vi "Utils - Convert1DImageToLVImage.vi"(6 "picture":picture, 8 "error in (no error)":errorcluster, 9 "1DImageData In":u8[](array[numeric]), 11 "Image Properties In":T1) -> (0 "error out":errorcluster, 1 "1DImageData Out":u8[](array[numeric]), 4 "new picture":picture)   [LabVIEW 2015]
doc: "Convert 1d U8 Image array to LabVIEW image. This VI supports only Mono8 image format."
uses:
  <vilib>/picture/picture.llb/Draw True-Color Pixmap.vi
  <vilib>/vision/NI_Vision_Development_Module.lvlib
  PRM/IMG_FORMAT/IMG_DATA_FORMAT.ctl
  xiImageManager/xiImageMng - Attributes.ctl
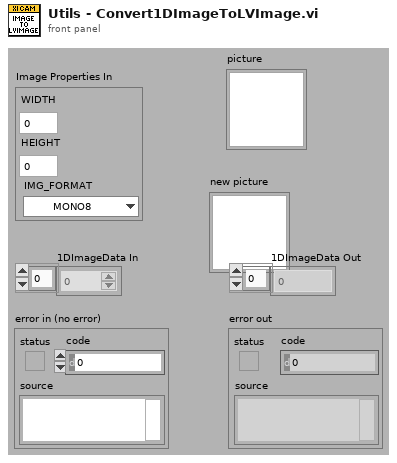
[diagram p1: front panel]
types:
  T1 = typedef "xiImageMng - Attributes.ctl" = cluster{"WIDTH":i32, "HEIGHT":i32, "IMG_FORMAT":T2}
  T2 = typedef "IMG_DATA_FORMAT.ctl" = enum16{"MONO8", "MONO16", "RGB24", "RGB32", "RGBPLANAR", "RAW8", "RAW16"}
  T3 = typedef "Image Type" = u32
  T4 = typedef "IMAQ Image.ctl" = refnum<image>
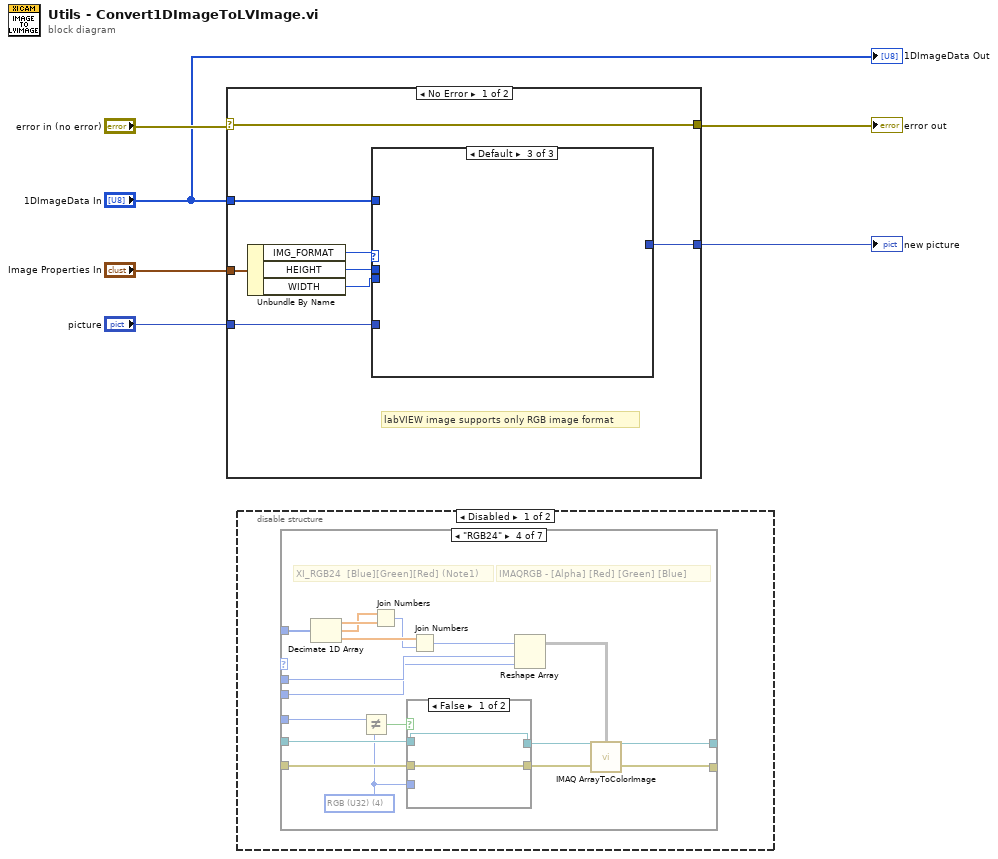
[diagram p0: block diagram]
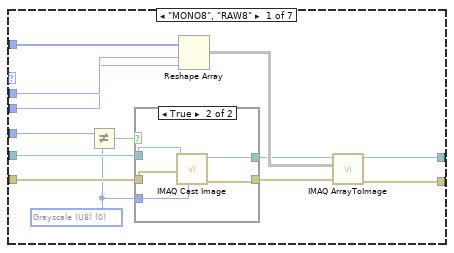
[diagram p2: hidden frame]
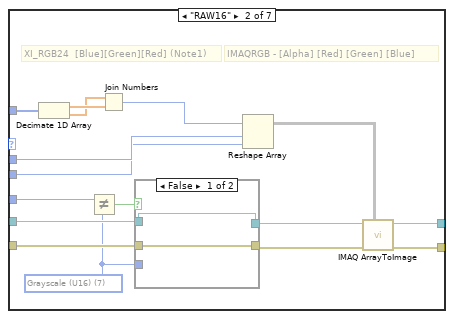
[diagram p4: hidden frame]
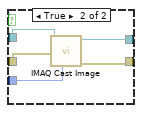
[diagram p5: hidden frame]
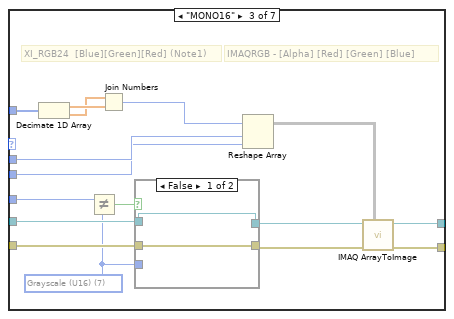
[diagram p6: hidden frame]
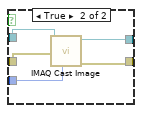
[diagram p7: hidden frame]
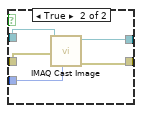
[diagram p8: hidden frame]
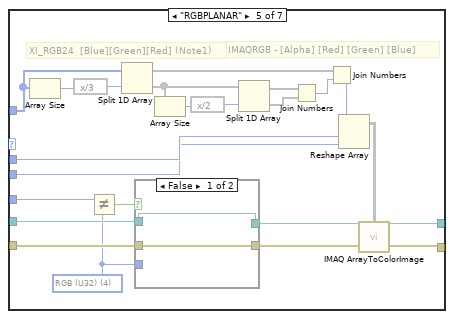
[diagram p9: hidden frame]
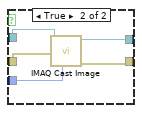
[diagram p10: hidden frame]
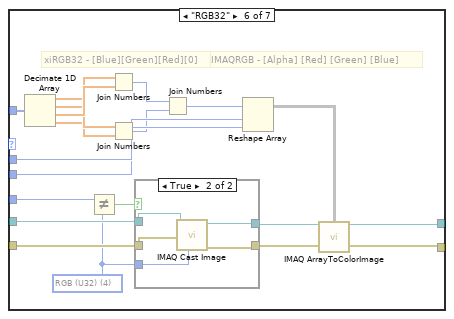
[diagram p11: hidden frame]
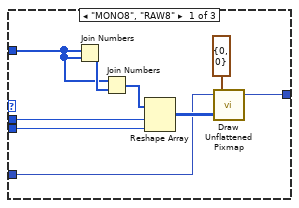
[diagram p15: hidden frame]
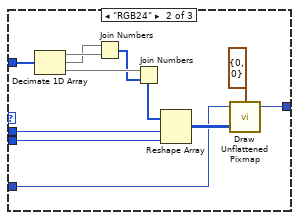
[diagram p16: hidden frame]
diagram:
  n1 = case shown="No Error" "error in (no error)" {
    selector: "error in (no error)" -> [w10 w36]
    tunnel: [w10 w36] -> w5
    tunnel: "1DImageData In" -> [w14 _]
    tunnel: [w13 _] -> w3
    tunnel: "Image Properties In" -> [w9 _]
    tunnel: "picture" -> [w8 _]
    frame No Error {
      # "labVIEW image supports only RGB image format"
      n2 = Unbundle By Name(w9) -> ("IMG_FORMAT"=w7:T2, "HEIGHT"=w12:i32, "WIDTH"=w11:i32)
      n3 = case shown="Default" w7 {
        tunnel: w14 -> [w19 w25 _]
        tunnel: [w18 w33 _] -> w13
        tunnel: w12 -> [w17 w32 _]
        tunnel: w11 -> [w16 w31 _]
        tunnel: w8 -> [w15 w30 _]
        frame "MONO8", "RAW8" {
          n4 = Join Numbers(hi=w19, lo=w19) -> ((hi.lo)=w20:u16[])
          n5 = Join Numbers(hi=w19, lo=w20) -> ((hi.lo)=w22:u32[])
          n6 = Reshape Array(w22, w17, w16) -> (w23:u32[][])
          n7 = call-poly <vilib>:"Draw Unflattened Pixmap.vi"("picture"=w15, "top left point(0, 0)"=cluster{"x":i16, "y":i16} {"x"=0, "y"=0}, "data (RGB format)"=w23) -> ("new picture"=w18:picture)  [unwired: 6 in]
        }
        frame "RGB24" {
          n8 = Decimate 1D Array(w25) -> (w28:u8[], w27:u8[], w29:u8[])
          n9 = Join Numbers(hi=w27, lo=w28) -> ((hi.lo)=w26:u16[])
          n10 = Join Numbers(hi=w29, lo=w26) -> ((hi.lo)=w24:u32[])
          n11 = Reshape Array(w24, w32, w31) -> (w35:u32[][])
          n12 = call-poly <vilib>:"Draw Unflattened Pixmap.vi"("picture"=w30, "top left point(0, 0)"=cluster{"x":i16, "y":i16} {"x"=0, "y"=0}, "data (RGB format)"=w35) -> ("new picture"=w33:picture)  [unwired: 6 in]
        }
        frame Default {
        }
      }
    }
    frame Error {
    }
  }
  "error out" <- w5
  "new picture" <- w3
  n13 = disable-structure shown="Disabled" {
    frame Disabled {
      n14 = case shown="\"RGB24\"" {
        selector: _ -> [_ _ _ _ _ _ _]
        tunnel: _ -> [w49 w63 w86 w104 w136 w170 _]
        tunnel: _ -> [w48 w72 w95 w120 w150 w177 _]
        tunnel: _ -> [w47 w71 w94 w119 w149 w176 _]
        tunnel: _ -> [w43 w67 w90 w115 w145 w172 w185]
        tunnel: _ -> [w46 w70 w93 w118 w148 w175 _]
        tunnel: _ -> [w44 w68 w91 w116 w146 w173 w186]
        tunnel: [w38 w61 w84 w110 w140 w166 w186] -> _
        tunnel: [w37 w60 w83 w109 w139 w165 w185] -> _
        frame "MONO8", "RAW8" {
          w42 = T3 0 items=["Grayscale (U8)", "Grayscale (I16)", "Grayscale (SGL)", "Complex (CSG)", "RGB (U32)", "HSL (U32)", "RGB (U64)", "Grayscale (U16)"] ("Image Type")
          n15 = Not Equal?(x=w46, y=w42) -> (x != y?=w45:bool)
          n16 = case shown="True" w45 {
            tunnel: w44 -> [w50 w56]
            tunnel: w43 -> [w51 w55]
            tunnel: w42 -> [_ w54]
            tunnel: [w50 w53] -> w40
            tunnel: [w51 w52] -> w39
            frame False {
            }
            frame True {
              n17 = call "IMAQ Cast Image"("Image Type"=w54, "error in (no error)"=w55, "Image Src"=w56) -> ("error out"=w52:errorcluster, "Image Dst Out"=w53:T4)  [unwired: 7 in]
            }
          }
          n18 = Reshape Array(w49, w48, w47) -> (w41:void[][])
          n19 = call "IMAQ ArrayToImage"("error in (no error)"=w39, "Image Pixels (U8)"=w41, "Image"=w40) -> ("error out"=w37:errorcluster, "Image Out"=w38:T4)  [unwired: 7 in]
        }
        frame "RAW16" {
          w66 = T3 7 items=["Grayscale (U8)", "Grayscale (I16)", "Grayscale (SGL)", "Complex (CSG)", "RGB (U32)", "HSL (U32)", "RGB (U64)", "Grayscale (U16)"] ("Image Type")
          # "IMAQRGB - [Alpha] [Red] [Green] [Blue]"
          # "XI_RGB24\t [Blue][Green][Red] (Note1)"
          n20 = Decimate 1D Array(w63) -> (w65:dbl[], w64:dbl[])
          n21 = Not Equal?(x=w70, y=w66) -> (x != y?=w69:bool)
          n22 = Join Numbers(hi=w64, lo=w65) -> ((hi.lo)=w62:u32)
          n23 = case shown="False" w69 {
            tunnel: w68 -> [w73 w79]
            tunnel: w67 -> [w74 w78]
            tunnel: w66 -> [_ w77]
            tunnel: [w73 w76] -> w58
            tunnel: [w74 w75] -> w59
            frame False {
            }
            frame True {
              n24 = call "IMAQ Cast Image"("Image Type"=w77, "error in (no error)"=w78, "Image Src"=w79) -> ("error out"=w75:errorcluster, "Image Dst Out"=w76:T4)  [unwired: 7 in]
            }
          }
          n25 = Reshape Array(w62, w72, w71) -> (w57:void[][])
          n26 = call "IMAQ ArrayToImage"("Image Pixels (U16)"=w57, "error in (no error)"=w59, "Image"=w58) -> ("error out"=w60:errorcluster, "Image Out"=w61:T4)  [unwired: 7 in]
        }
        frame "MONO16" {
          w89 = T3 7 items=["Grayscale (U8)", "Grayscale (I16)", "Grayscale (SGL)", "Complex (CSG)", "RGB (U32)", "HSL (U32)", "RGB (U64)", "Grayscale (U16)"] ("Image Type")
          # "IMAQRGB - [Alpha] [Red] [Green] [Blue]"
          # "XI_RGB24\t [Blue][Green][Red] (Note1)"
          n27 = Decimate 1D Array(w86) -> (w88:dbl[], w87:dbl[])
          n28 = Not Equal?(x=w93, y=w89) -> (x != y?=w92:bool)
          n29 = Join Numbers(hi=w87, lo=w88) -> ((hi.lo)=w85:u32)
          n30 = case shown="False" w92 {
            tunnel: w91 -> [w96 w102]
            tunnel: w90 -> [w97 w101]
            tunnel: w89 -> [_ w100]
            tunnel: [w96 w99] -> w81
            tunnel: [w97 w98] -> w82
            frame False {
            }
            frame True {
              n31 = call "IMAQ Cast Image"("Image Type"=w100, "error in (no error)"=w101, "Image Src"=w102) -> ("error out"=w98:errorcluster, "Image Dst Out"=w99:T4)  [unwired: 7 in]
            }
          }
          n32 = Reshape Array(w85, w95, w94) -> (w80:void[][])
          n33 = call "IMAQ ArrayToImage"("Image Pixels (U16)"=w80, "error in (no error)"=w82, "Image"=w81) -> ("error out"=w83:errorcluster, "Image Out"=w84:T4)  [unwired: 7 in]
        }
        frame "RGB24" {
          w114 = T3 4 items=["Grayscale (U8)", "Grayscale (I16)", "Grayscale (SGL)", "Complex (CSG)", "RGB (U32)", "HSL (U32)", "RGB (U64)", "Grayscale (U16)"] ("Image Type")
          # "IMAQRGB - [Alpha] [Red] [Green] [Blue]"
          # "XI_RGB24\t [Blue][Green][Red] (Note1)"
          n34 = Decimate 1D Array(w104) -> (w107:dbl[], w106:dbl[], w108:dbl[])
          n35 = Not Equal?(x=w118, y=w114) -> (x != y?=w117:bool)
          n36 = Join Numbers(hi=w106, lo=w107) -> ((hi.lo)=w105:u32)
          n37 = case shown="False" w117 {
            tunnel: w116 -> [w121 w127]
            tunnel: w115 -> [w122 w126]
            tunnel: w114 -> [_ w125]
            tunnel: [w121 w124] -> w113
            tunnel: [w122 w123] -> w111
            frame False {
            }
            frame True {
              n38 = call "IMAQ Cast Image"("Image Type"=w125, "error in (no error)"=w126, "Image Src"=w127) -> ("error out"=w123:errorcluster, "Image Dst Out"=w124:T4)  [unwired: 7 in]
            }
          }
          n39 = Join Numbers(hi=w108, lo=w105) -> ((hi.lo)=w103:u64)
          n40 = Reshape Array(w103, w120, w119) -> (w112:void[][])
          n41 = call "IMAQ ArrayToColorImage"("Image Pixels (U32)"=w112, "Image"=w113, "error in (no error)"=w111) -> ("Image Out"=w110:T4, "error out"=w109:errorcluster)  [unwired: 2 in]
        }
        frame "RGBPLANAR" {
          w144 = T3 4 items=["Grayscale (U8)", "Grayscale (I16)", "Grayscale (SGL)", "Complex (CSG)", "RGB (U32)", "HSL (U32)", "RGB (U64)", "Grayscale (U16)"] ("Image Type")
          # "IMAQRGB - [Alpha] [Red] [Green] [Blue]"
          # "XI_RGB24\t [Blue][Green][Red] (Note1)"
          n42 = Array Size(array=w136) -> (size(s)=w137:i32)
          n43 = expression code="x/3"(w137) -> (w138:i32)
          n44 = Not Equal?(x=w148, y=w144) -> (x != y?=w147:bool)
          n45 = Split 1D Array(array=w136, index=w138) -> (first subarray=w135:void[], second subarray=w132:void[])
          n46 = case shown="False" w147 {
            tunnel: w146 -> [w151 w157]
            tunnel: w145 -> [w152 w156]
            tunnel: w144 -> [_ w155]
            tunnel: [w151 w154] -> w143
            tunnel: [w152 w153] -> w141
            frame False {
            }
            frame True {
              n47 = call "IMAQ Cast Image"("Image Type"=w155, "error in (no error)"=w156, "Image Src"=w157) -> ("error out"=w153:errorcluster, "Image Dst Out"=w154:T4)  [unwired: 7 in]
            }
          }
          n48 = Array Size(array=w132) -> (size(s)=w134:i32)
          n49 = expression code="x/2"(w134) -> (w133:i32)
          n50 = Split 1D Array(array=w132, index=w133) -> (first subarray=w131:void[], second subarray=w130:void[])
          n51 = Join Numbers(hi=w131, lo=w130) -> ((hi.lo)=w129:u32)
          n52 = Join Numbers(hi=w135, lo=w129) -> ((hi.lo)=w128:u64)
          n53 = Reshape Array(w128, w150, w149) -> (w142:void[][])
          n54 = call "IMAQ ArrayToColorImage"("Image Pixels (U32)"=w142, "Image"=w143, "error in (no error)"=w141) -> ("Image Out"=w140:T4, "error out"=w139:errorcluster)  [unwired: 2 in]
        }
        frame "RGB32" {
          w171 = T3 4 items=["Grayscale (U8)", "Grayscale (I16)", "Grayscale (SGL)", "Complex (CSG)", "RGB (U32)", "HSL (U32)", "RGB (U64)", "Grayscale (U16)"] ("Image Type")
          # "IMAQRGB - [Alpha] [Red] [Green] [Blue]"
          # "xiRGB32 - [Blue][Green][Red][0]"
          n55 = Decimate 1D Array(w170) -> (w160:dbl[], w161:dbl[], w162:dbl[], w158:dbl[])
          n56 = Not Equal?(x=w175, y=w171) -> (x != y?=w174:bool)
          n57 = Join Numbers(hi=w158, lo=w162) -> ((hi.lo)=w164:u32)
          n58 = Join Numbers(hi=w161, lo=w160) -> ((hi.lo)=w163:u32)
          n59 = case shown="True" w174 {
            tunnel: w173 -> [w178 w184]
            tunnel: w172 -> [w179 w183]
            tunnel: w171 -> [_ w182]
            tunnel: [w178 w181] -> w169
            tunnel: [w179 w180] -> w167
            frame False {
            }
            frame True {
              n60 = call "IMAQ Cast Image"("Image Type"=w182, "error in (no error)"=w183, "Image Src"=w184) -> ("error out"=w180:errorcluster, "Image Dst Out"=w181:T4)  [unwired: 7 in]
            }
          }
          n61 = Join Numbers(hi=w164, lo=w163) -> ((hi.lo)=w159:u64)
          n62 = Reshape Array(w159, w177, w176) -> (w168:void[][])
          n63 = call "IMAQ ArrayToColorImage"("Image Pixels (U32)"=w168, "Image"=w169, "error in (no error)"=w167) -> ("Image Out"=w166:T4, "error out"=w165:errorcluster)  [unwired: 2 in]
        }
        frame Default {
        }
      }
    }
    frame Enabled {
    }
  }
  "1DImageData Out" <- "1DImageData In"
